vi "fwhm test.vi"() -> ()   [LabVIEW 2016]
uses:
  <vilib>/Analysis/NI_AALPro.lvlib
panel:
  out "fwhm":i32
  out "location":dbl
  out "peak":dbl
  in  "stop":bool
  out "MCA Histograms":u32[][](graph)
  in  "channel":string(combo)
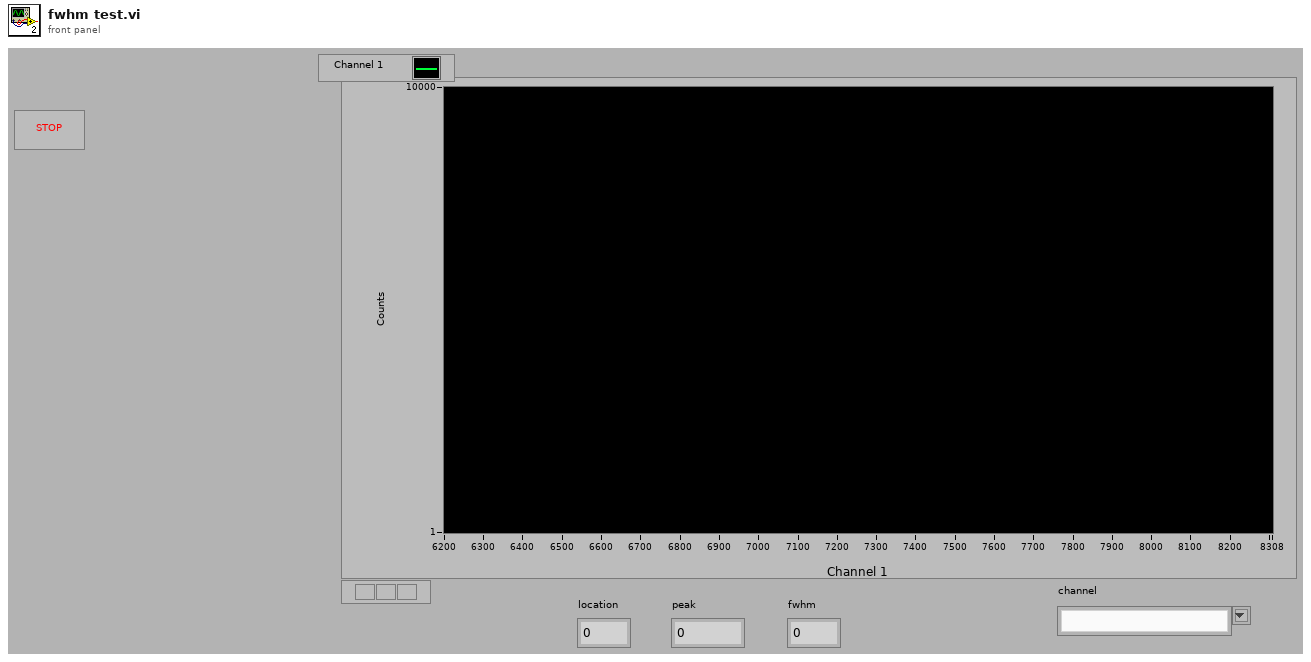
[diagram p1: front panel]
types:
  T1 = typedef "LVPoint32TypeDef.ctl" = cluster{"Horizontal":i32, "Vertical":i32}
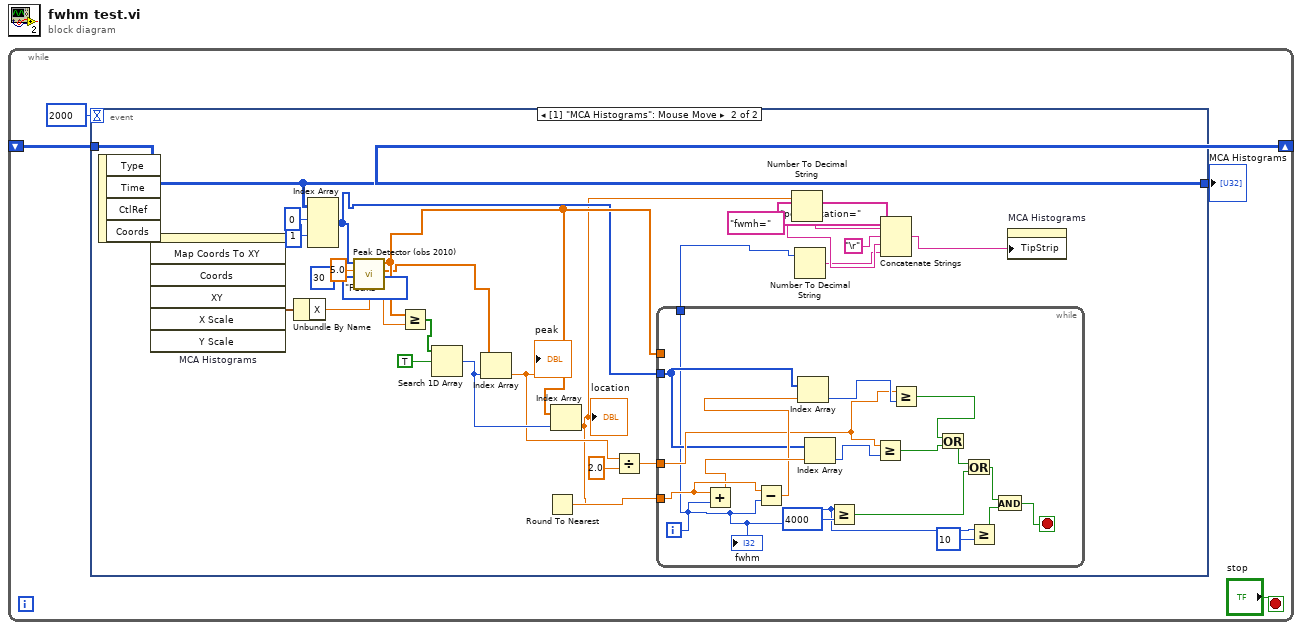
[diagram p0: block diagram]
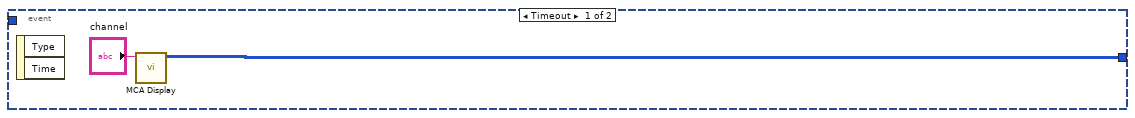
[diagram p2: hidden frame]
diagram:
  n1 = while {
    shift-right: [w3] -> _
    shift-left: _ -> [w1]
    stop <- "stop" stop-if-true
    n2 = event shown="[1] \"MCA Histograms\": Mouse Move" {
      selector: _ -> [_ _]
      dyn-events: _ -> [_ _]
      timeout: 2000 -> [_ _]
      tunnel: [w5 w31] -> w3
      tunnel: w1 -> [_ w31]
      event Timeout {
        n3 = event-data() -> ()  [unwired: 1 in, 2 out]
        n4 = call "MCA Display.vi"("channel"="channel") -> ("MCA Histograms"=w5:u32[][])  [unwired: 7 in, 3 out]
      }
      event "MCA Histograms": Mouse Move {
        n5 = event-data() -> ("Coords"=w33:T1)  [unwired: 1 in, 3 out]
        n6 = invoke on="MCA Histograms" class="WFGraph (strict)" method="Map Coords To XY"("Coords"=w33) -> ("XY"=w32:cluster{"X":dbl, "Y":dbl})  [unwired: 6 in, 6 out]
        n7 = Unbundle By Name(w32) -> ("X"=w27:dbl)
        n8 = Index Array(array=w31, index (row) #1=0 ("index (row)"), index (row) #2=1 ("disabled index (col)")) -> (element #1=w15:u32[])  [unwired: 2 in, 1 out]
        n9 = call <vilib>:"Peak Detector (obs 2010).vi"("peaks/valleys"=enum32{"Peaks", "Valleys"}."Peaks", "width"=30, "threshold"=5.0, "X"=w15) -> ("Amplitudes"=w20:dbl[], "Locations"=w21:dbl[])  [unwired: 3 in, 3 out]
        n10 = Greater Or Equal?(x=w21, y=w27) -> (x >= y?=w26:bool[])
        n11 = Search 1D Array(1D array=w26, element=TRUE) -> (index of element=w24:i32)  [unwired: 1 in]
        n12 = Index Array(array=w20, index=w24) -> (element=w17:dbl)
        "peak" <- w17
        n13 = Index Array(array=w21, index=w24) -> (element=w13:dbl)
        "location" <- w13
        n14 = Round To Nearest(number=w13) -> (nearest integer value=w18:dbl)
        n15 = Divide(x=w17, y=2.0) -> (x/y=w22:dbl)
        n16 = while {
          tunnel: w18 -> [w50]
          tunnel: w22 -> [w40]
          tunnel: w21 -> [_]
          tunnel: w15 -> [w35]
          tunnel: [w34] -> w8
          i -> [w34]
          stop <- w36 stop-if-true
          n17 = Add(x=w50, y=w34) -> (x+y=w49:dbl)
          n18 = Subtract(x=w50, y=w34) -> (x-y=w48:dbl)
          n19 = Index Array(array=w35, index=w48) -> (element=w42:u32)
          n20 = Index Array(array=w35, index=w49) -> (element=w41:u32)
          n21 = Greater Or Equal?(x=w34, y=4000) -> (x >= y?=w44:bool)
          n22 = Greater Or Equal?(x=w40, y=w41) -> (x >= y?=w43:bool)
          n23 = Greater Or Equal?(x=w40, y=w42) -> (x >= y?=w47:bool)
          n24 = Or(x=w47, y=w43) -> (x .or. y?=w45:bool)
          n25 = Or(x=w45, y=w44) -> (x .or. y?=w39:bool)
          n26 = Greater Or Equal?(x=w34, y=10) -> (x >= y?=w37:bool)
          n27 = And(x=w39, y=w37) -> (x .and. y?=w36:bool)
          "fwhm" <- w34
        }
        n28 = Number To Decimal String(number=w13) -> (decimal integer string=w12:string)  [unwired: 1 in]
        n29 = Number To Decimal String(number=w8) -> (decimal integer string=w9:string)  [unwired: 1 in]
        n30 = Concatenate Strings("peak location=" ("Tip Strip"), w12, "\r", "fwmh=" ("Tip Strip"), w9) -> (w7:string)
        n31 = property on="MCA Histograms" class="WFGraph (strict)"("TipStrip"=w7) -> ()  [unwired: 2 in, 2 out]
      }
    }
    "MCA Histograms" <- w3
  }
